vi "LEIN CMD create STAT.vi"(0 "SID":u8, 7 "STAT ID":u8, 9 "STAT Part":u8, 11 "error in (no error)":errorcluster) -> (8 "CMD":T1={"SID"=0, "ANF"=FALSE, "CMD"=enum."TASK", "DATA"=[]}, 15 "error out":errorcluster)   [LabVIEW 2011]
uses:
  Defenitions/LEIN CMD Cluster.ctl
  Defenitions/LEIN CMD List.ctl
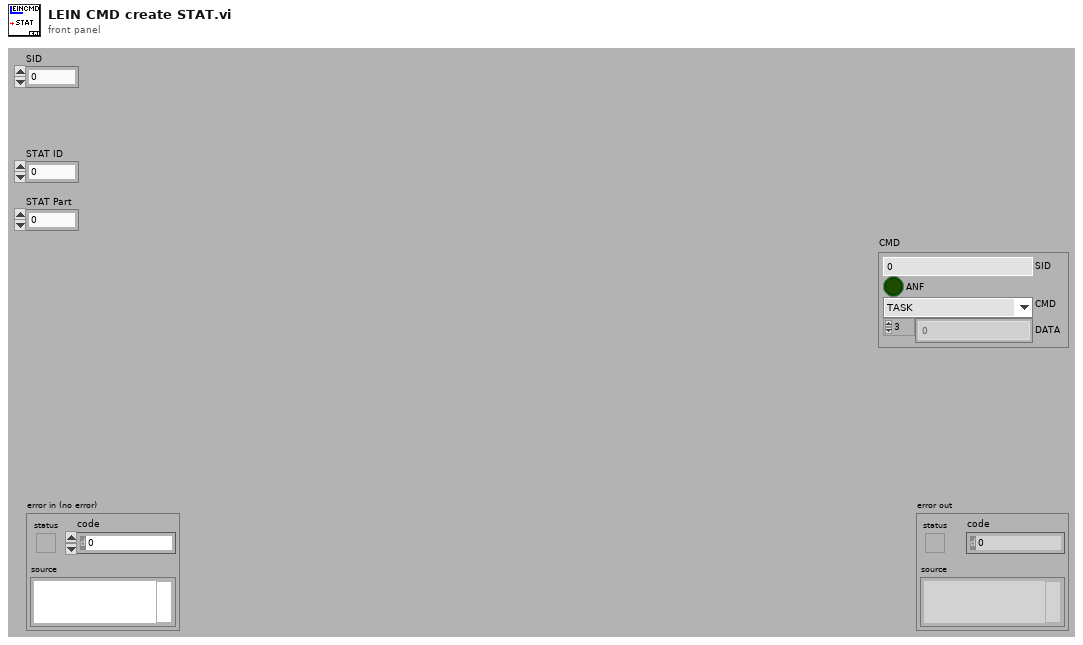
[diagram p1: front panel]
types:
  T1 = typedef "LEIN CMD Cluster.ctl" = cluster{"SID":u8, "ANF":bool, "CMD":T2, "DATA":u8[]}
  T2 = typedef "LEIN CMD List.ctl" = enum8{"ACTI", "TASK", "RES0", "STAT", "RES1", "RES2", "RES3", "USER"}
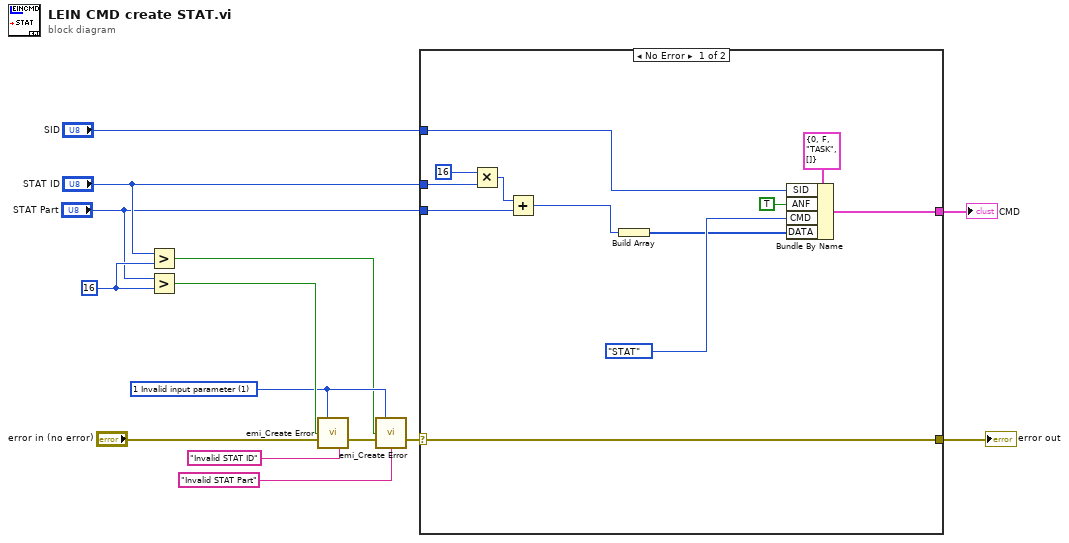
[diagram p0: block diagram]
diagram:
  w12 = 1 items=["0 No Error"=0, "1 Invalid input parameter"=1, "6 Generic file IO "=6, "7 File not Found"=7, "35 Generic Pring Error"=35, "37 Device not Found"=37, "39 Device Unit Error"=39, "40 Could fot Open Device"=40, "42 Generic Error"=42, "52 Unknown Message"=52, "98 Bad File type"=98, "99 Bad File Version"=99, "100 Bad Data in File"=100, "1018 Unspecefied Error"=1018, "1041 Incorrect Password"=1041, "1043 Feature not in this version"=1043, "1109 Unsuported Data type"=1109, "1444 Did not close sucessfully"=1444] ("Error Code")
  w14 = u8 16 ("y")
  n1 = Greater?(x="STAT ID", y=w14) -> (0:w11:bool)
  n2 = Greater?(x="STAT Part", y=w14) -> (0:w13:bool)
  n3 = call "emi_Create Error.vi"("Error Code"=w12, "Error(T)"=w13, "error in (no error)"="error in (no error)", "Append String(\"\")"="Invalid STAT ID" ("Append String(\"\")")) -> ("error out"=w9:errorcluster)  [unwired: 11 in]
  n4 = call "emi_Create Error.vi"("Error Code"=w12, "Error(T)"=w11, "error in (no error)"=w9, "Source String(\"\")"="Invalid STAT Part" ("Source String(\"\")")) -> ("error out"=w6:errorcluster)  [unwired: 11 in]
  n5 = case shown="No Error" w6 {
    selector: w6 -> [w26 w27]
    tunnel: [w26 w27] -> w5
    tunnel: "STAT ID" -> [w25 _]
    tunnel: "STAT Part" -> [w22 _]
    tunnel: [w20 _] -> w2
    tunnel: "SID" -> [w19 _]
    frame No Error {
      n6 = Multiply(x=u8 16, y=w25) -> (x*y=w23:u8)
      n7 = Add(x=w23, y=w22) -> (x+y=w16:u8)
      n8 = Build Array(w16) -> (w15:u8[])
      n9 = Bundle By Name(cluster=T1 {"SID"=0, "ANF"=FALSE, "CMD"=enum."TASK", "DATA"=[]} ("CMD"), "SID"=w19, "ANF"=TRUE, "CMD"=LEIN_CMD_List."STAT", "DATA"=w15) -> (w20:T1)
    }
    frame Error {
    }
  }
  "error out" <- w5
  "CMD" <- w2
